vi "Get SMO Database Paths.vi"(5 "getAll Cluster":variant, 7 "Paths":string="llab_038:d000(TEST_TABLE--Temperature(Kelvin))\nllab_038:d002(TEST_TABLE--voltage 2(volts))\nllab_038:b000(TEST_TABLE--ON?())\nllab_038:v001(TEST_TABLE--sample())", 8 "error in (no error)":errorcluster, 11 "Inst.Krohn-Hite-7008 in":refnum<class "Inst.Krohn-Hite-7008.lvclass">) -> (0 "error out":errorcluster, 2 "Paths":string, 3 "Inst.Krohn-Hite-7008 out":refnum<class "Inst.Krohn-Hite-7008.lvclass">)   [LabVIEW 2019, in "Inst.KH7008.lvlib" / "Inst.Krohn-Hite-7008.lvclass"]
uses:
  Inst.Krohn-Hite-7008.lvclass
  Typedefs/Inst.Krohn-Hite-7008.getAll--Cluster.ctl
  KH7008/typedefs/allChannelProperties--Array.ctl
  KH7008/typedefs/channelProperties--Cluster.ctl
  KH7008/typedefs/channel--numeric.ctl
  KH7008/typedefs/gain--enum.ctl
  KH7008/typedefs/Input--Enum.ctl
  KH7008/typedefs/shunt--enum.ctl
  KH7008/typedefs/couple--Enum.ctl
  KH7008/typedefs/Filter--Enum.ctl
  Typedefs/Inst.Krohn-Hite-7008.device--Cluster.ctl
  Typedefs/getAllChannelsDatabase--Cluster.ctl
  <userlib>/LevyLab/Instrument Framework/Instrument Types/Amplifier/Instrument.Amplifier.lvclass
  <userlib>/LevyLab/LV-Data/LV-Data.PG/LV-Data.PGSQL.lvclass
  <userlib>/LevyLab/LV-Data/LV-Data.PG/API/Write Variable (one-row).vi
  KH7008/KH7008.lvlib
panel:
  in  "getAll":T1 {"allChannelProperties"."channel" min=1 max=8 step=1}
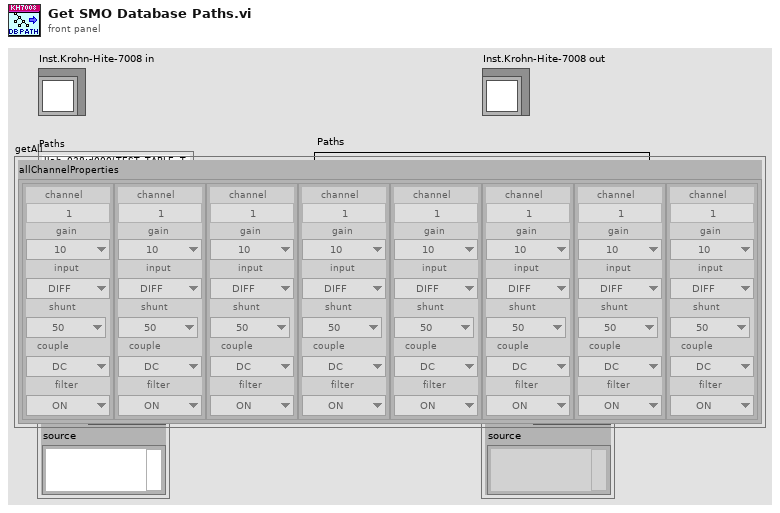
[diagram p1: front panel]
types:
  T1 = typedef "Inst.KH7008.lvlib/Inst.Krohn-Hite-7008.lvclass/Inst.Krohn-Hite-7008.getAll--Cluster.ctl" = cluster{"allChannelProperties":T2}
  T2 = typedef "KH7008.lvlib/allChannelProperties--Array.ctl" = T3[]
  T3 = typedef "KH7008.lvlib/channelProperties--Cluster.ctl" = cluster{"channel":T4, "gain":T5, "input":T6, "shunt":T7, "couple":T8, "filter":T9}
  T4 = typedef "KH7008.lvlib/channel--numeric.ctl" = u16
  T5 = typedef "KH7008.lvlib/gain--enum.ctl" = enum16{"1", "10", "100", "1000"}
  T6 = typedef "KH7008.lvlib/input--enum.ctl" = enum16{"OFF", "SE+", "SE-", "DIFF"}
  T7 = typedef "KH7008.lvlib/shunt--enum.ctl" = enum16{"Open", "50", "500", "5k", "50k", "10M"}
  T8 = typedef "KH7008.lvlib/couple--enum.ctl" = enum16{"AC", "DC"}
  T9 = typedef "KH7008.lvlib/filter--enum.ctl" = enum16{"OFF", "ON"}
  T10 = typedef "Inst.KH7008.lvlib/Inst.Krohn-Hite-7008.lvclass/getAllChannelsDatabase--Cluster.ctl" = cluster{"channel":u32, "gain":string, "input":string, "shunt":string, "couple":string, "filter":string, "model":string, "device_id":string}
  T11 = typedef "Inst.KH7008.lvlib/Inst.Krohn-Hite-7008.lvclass/Inst.Krohn-Hite-7008.device--Cluster.ctl" = cluster{"model":string, "device_id":string}
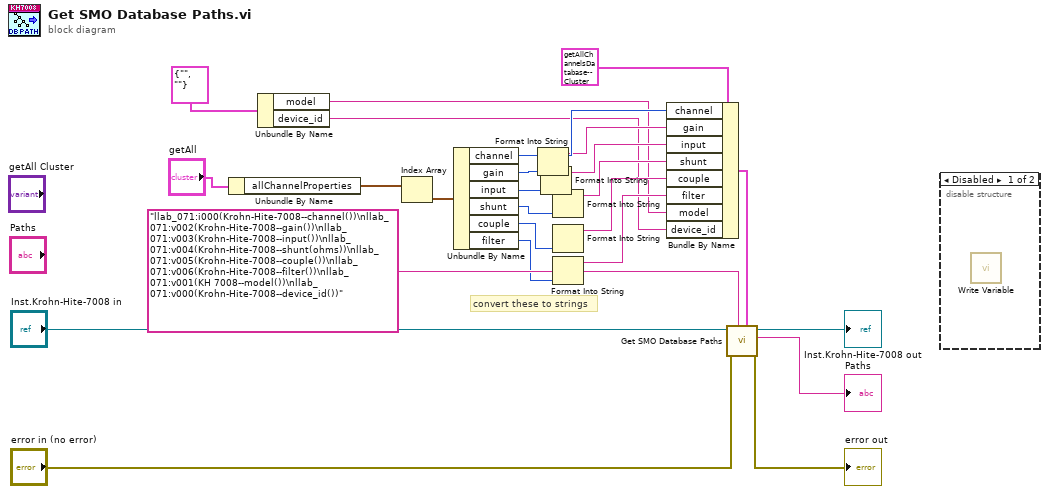
[diagram p0: block diagram]
diagram:
  # "convert these to strings"
  n1 = Unbundle By Name("getAll") -> ("allChannelProperties"=w18:T2)
  n2 = Unbundle By Name(T11 {"model"="", "device_id"=""} ("Device")) -> ("model"=w2:string, "device_id"=w1:string)
  n3 = Index Array(array=w18) -> (element=w17:T3)  [unwired: 1 in]
  n4 = Unbundle By Name(w17) -> ("channel"=w13:T4, "gain"=w12:T5, "input"=w10:T6, "shunt"=w9:T7, "couple"=w8:T8, "filter"=w7:T9)
  n5 = Format Into String(w12) -> (resulting string=w11:string)  [unwired: 3 in, 1 out]
  n6 = Format Into String(w10) -> (resulting string=w6:string)  [unwired: 3 in, 1 out]
  n7 = Format Into String(w9) -> (resulting string=w5:string)  [unwired: 3 in, 1 out]
  n8 = Format Into String(w8) -> (resulting string=w4:string)  [unwired: 3 in, 1 out]
  n9 = Format Into String(w7) -> (resulting string=w3:string)  [unwired: 3 in, 1 out]
  n10 = Bundle By Name(cluster=T10 {"channel"=8, "gain"="1", "input"="OFF", "shunt"="Open", "couple"="DC", "filter"="ON", "model"="", "device_id"=""} ("getChannelResponse"), "channel"=w13, "gain"=w11, "input"=w6, "shunt"=w5, "couple"=w4, "filter"=w3, "model"=w2, "device_id"=w1) -> (w16:T10)
  n11 = call-parent "Get SMO Database Paths.vi"("getAll Cluster"=w16, "Default Paths"="llab_071:i000(Krohn-Hite-7008--channel())\nllab_071:v002(Krohn-Hite-7008--gain())\nllab_071:v003(Krohn-Hite-7008--input())\nllab_071:v004(Krohn-Hite-7008--shunt(ohms))\nllab_071:v005(Krohn-Hite-7008--couple())\nllab_071:v006(Krohn-Hite-7008--filter())\nllab_071:v001(KH 7008--model())\nllab_071:v000(Krohn-Hite-7008--device_id())" ("Paths"), "error in (no error)"="error in (no error)", "Instrument in"="Inst.Krohn-Hite-7008 in") -> ("error out"=→"error out":errorcluster, "Paths"=→"Paths":string, "Instrument out"=→"Inst.Krohn-Hite-7008 out":refnum<class "Inst.Krohn-Hite-7008.lvclass">)  [unwired: 5 in]
  n12 = disable-structure shown="Disabled" {
    frame Disabled {
      n13 = call-poly <userlib>:"Write Variable.vi"() -> ()  [unwired: 8 in, 4 out]
    }
    frame Enabled {
    }
  }
